vi "Decoder template.vi"(8 "error in (no error)":errorcluster, 10 "String":string) -> (0 "error out":errorcluster, 2 "Cluster":cluster{})   [LabVIEW 2020]
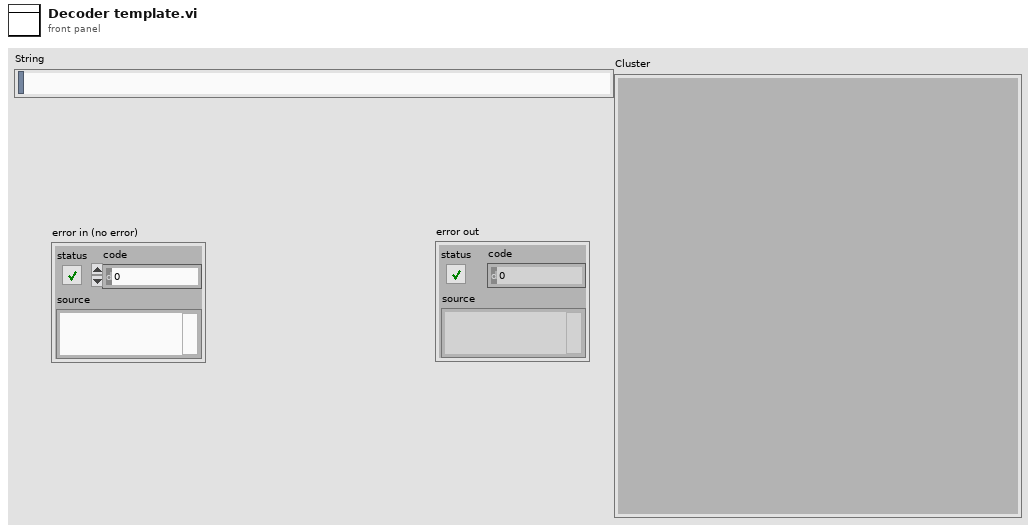
[diagram p1: front panel]
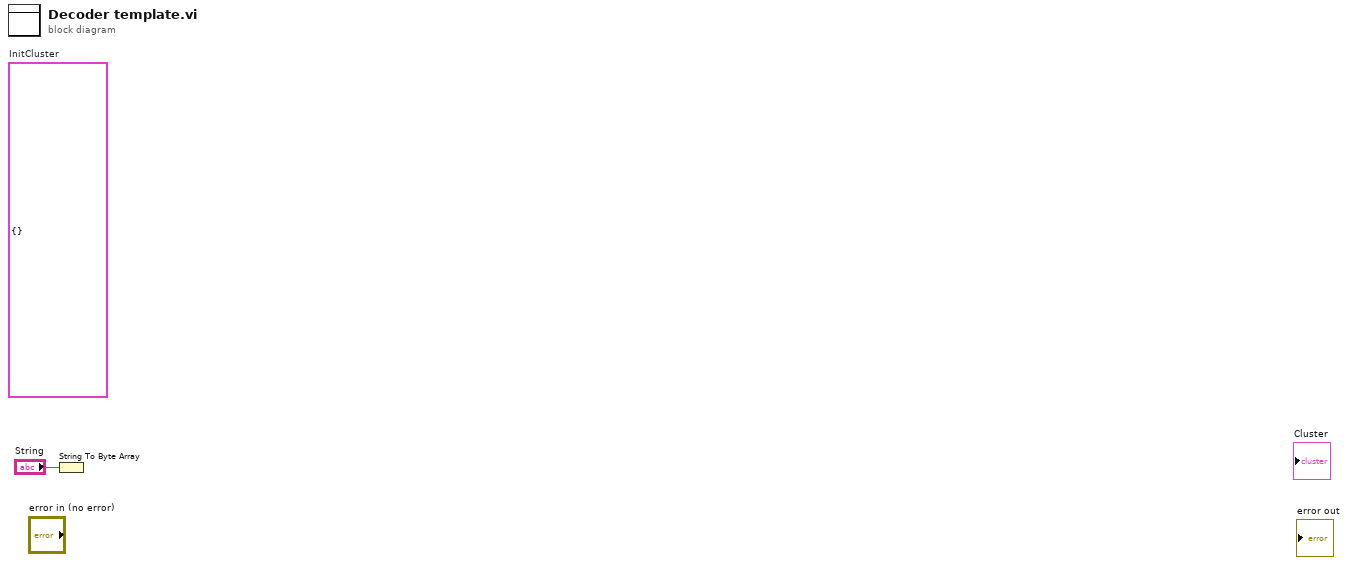
[diagram p0: block diagram]
diagram:
  (unwired) cluster{} {}  # InitCluster
  n1 = String To Byte Array(string="String") -> ()  [unwired: 1 out]
